vi "Donut Chart Test.vi"() -> ()   [LabVIEW 2016]
uses:
  Donut Chart/Donut Chart.xctl
panel:
  out "Donut Chart":T1(xcontrol)
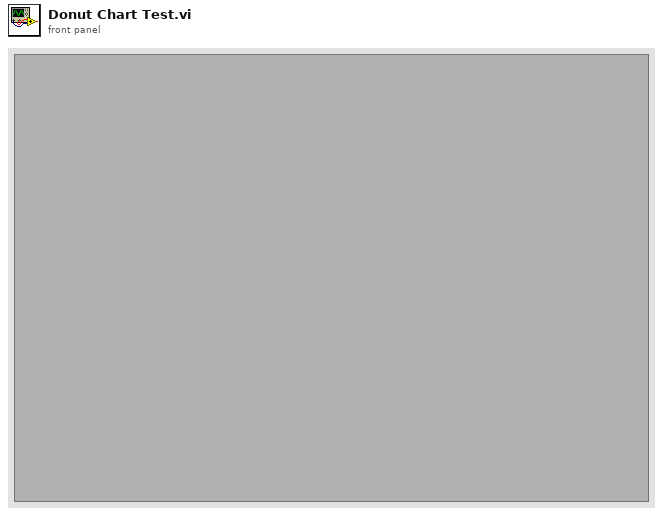
[diagram p1: front panel]
types:
  T1 = cluster{"Plot Title":string, "Plots":cluster{"Name":string, "Value":dbl, "Color":u32}[]}
  T2 = cluster{"Plot Title":string, "Plots":cluster{"Name":string, "Value":dbl, u32}[]}
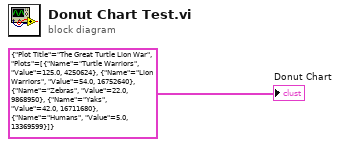
[diagram p0: block diagram]
diagram:
  "Donut Chart" <- T2 {"Plot Title"="The Great Turtle Lion War", "Plots"=[{"Name"="Turtle Warriors", "Value"=125.0, 4250624}, {"Name"="Lion Warriors", "Value"=54.0, 16752640}, {"Name"="Zebras", "Value"=22.0, 9868950}, {"Name"="Yaks", "Value"=42.0, 16711680}, {"Name"="Humans", "Value"=5.0, 13369599}]} ("Pie Chart")
